vi "Set New Frame Name.vi"(8 "error in (no error)":errorcluster, 10 "reference in":refnum<vi>, 11 "Setter Generator In":refnum<class "API VI Generator.lvclass">) -> (0 "error out":errorcluster, 2 "reference out":refnum<vi>, 3 "Setter Generator Out":refnum<class "API VI Generator.lvclass">)   [LabVIEW 2020, in "Method Generation.lvlib" / "API VI Generator.lvclass"]
uses:
  API VI Generator.lvclass
  API VI Generator.lvclass/API VI Generator.ctl
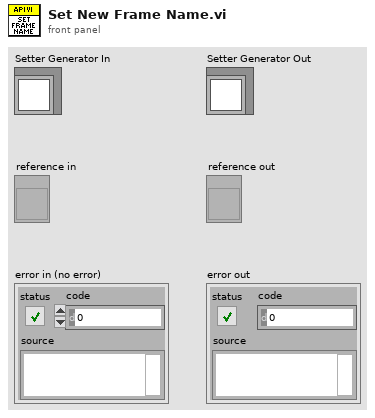
[diagram p1: front panel]
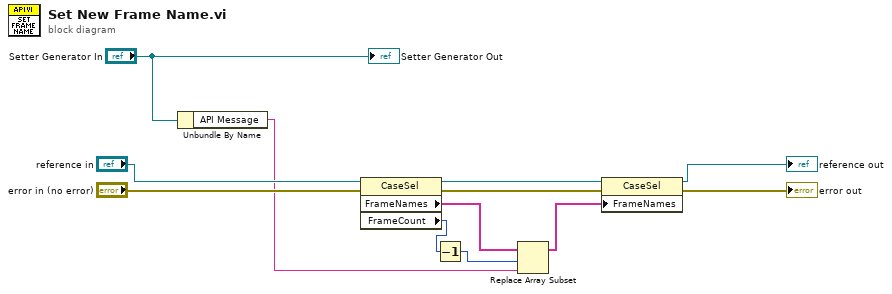
[diagram p0: block diagram]
diagram:
  n1 = Unbundle By Name("Setter Generator In") -> ("API Message"=w8:string)
  n2 = property class="CaseSel"(reference="reference in", error in="error in (no error)") -> (reference out=w3:refnum<vi>, error out=w12:errorcluster, "FrameNames"=w7:string[], "FrameCount"=w6:i32)
  n3 = Decrement(x=w6) -> (x-1=w5:i32)
  n4 = Replace Array Subset(array=w7, new element=w8, index=w5) -> (w1:string[])
  n5 = property class="CaseSel"(reference=w3, error in=w12, "FrameNames"=w1) -> (reference out=→"reference out":refnum<vi>, error out=→"error out":errorcluster)
  "Setter Generator Out" <- "Setter Generator In"
